vi "Parse_Raw_Response_HTTP.vi"(8 "error in (no error)":errorcluster, 11 "HTTP Response":string) -> (0 "error out":errorcluster, 1 "Headers":cluster{"Name":string, "Value":string}[](array[cluster]), 2 "Status Description":string, 3 "Status Code":string, 4 "Body":string)   [LabVIEW 2016, in "Response.lvclass"]
uses:
  Response.lvclass
panel:
  out "Protocol":string
  out "Status Line":string
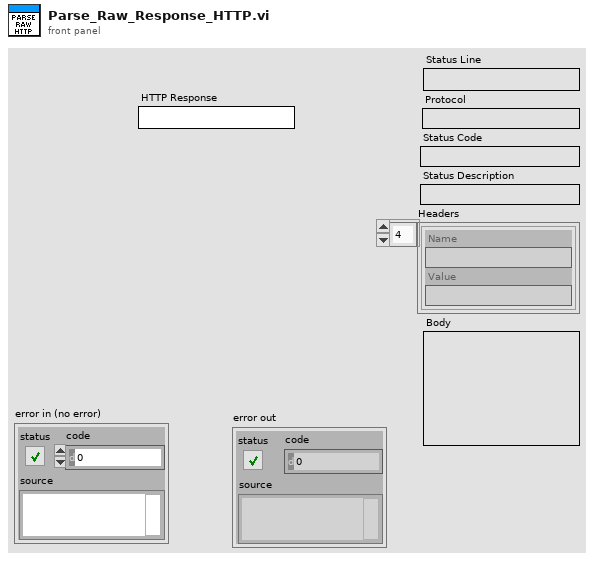
[diagram p1: front panel]
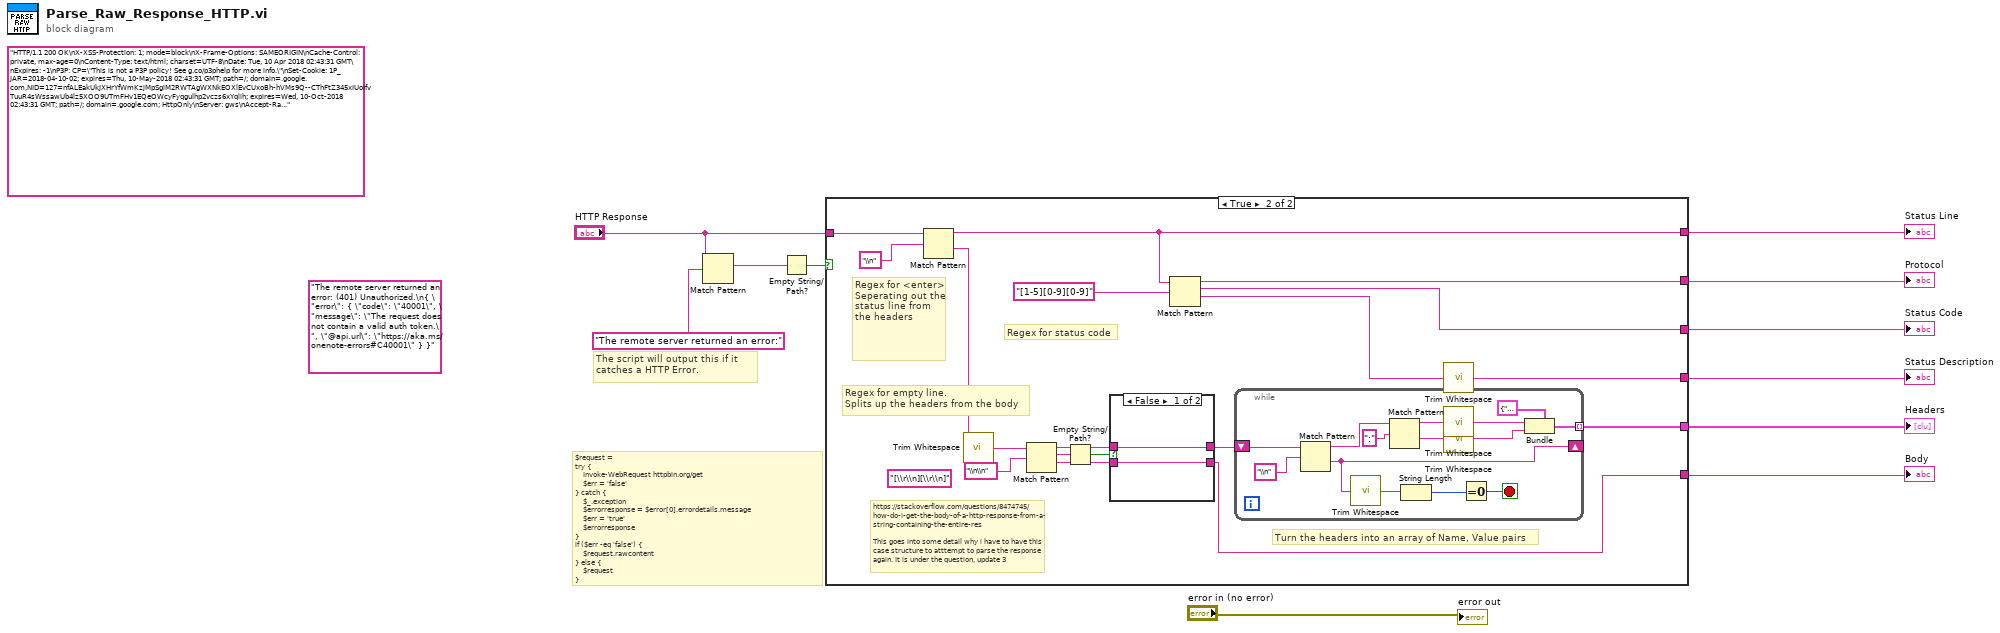
[diagram p0: block diagram]
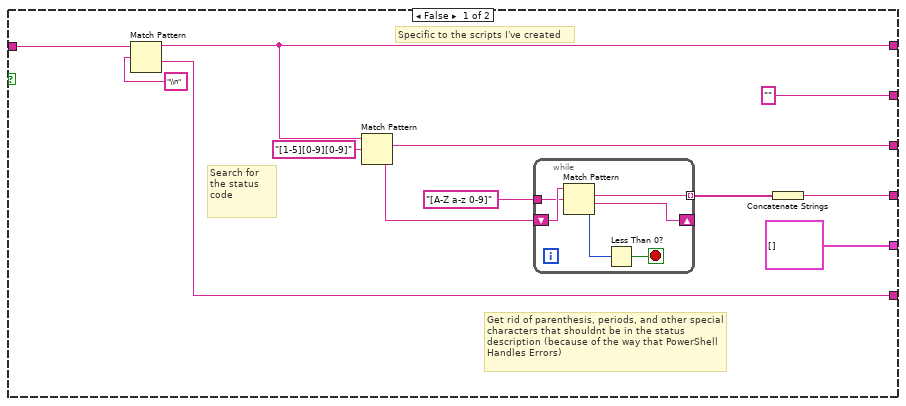
[diagram p2: hidden frame]
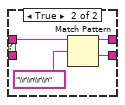
[diagram p3: hidden frame]
diagram:
  (unwired) "The remote server returned an error: (401) Unauthorized.\n{ \"error\": { \"code\": \"40001\", \"message\": \"The request does not contain a valid auth token.\", \"@api.url\": \"https://aka.ms/onenote-errors#C40001\" } }" ("string")
  (unwired) "HTTP/1.1 200 OK\nX-XSS-Protection: 1; mode=block\nX-Frame-Options: SAMEORIGIN\nCache-Control: private, max-age=0\nContent-Type: text/html; charset=UTF-8\nDate: Tue, 10 Apr 2018 02:43:31 GMT\nExpires: -1\nP3P: CP=\"This is not a P3P policy! See g.co/p3phelp for more info.\"\nSet-Cookie: 1P_JAR=2018-04-10-02; expires=Thu, 10-May-2018 02:43:31 GMT; path=/; domain=.google.com,NID=127=nfALEakUkJXHrYfWmKzjMpSgiM2RWTAgWXNkEOXlEvCUxoBh-hVMs9Q--CThFtZ345xIUoIfvTuuR4sWssawUb4lz5XOO9UTmFHv1EQeOWcyFyqgulhp2vczs6xYqlih; expires=Wed, 10-Oct-2018 02:43:31 GMT; path=/; domain=.google.com; HttpOnly\nServer: gws\nAccept-Ranges: none\nVary: Accept-Encoding\nTransfer-Encoding: chunked\n\n<!doctype html><html itemscope=\"\" itemtype=\"http://schema.org/WebPage\" lang=\"en\"><head><meta content=\"Search the world's information, including webpages, images, videos and more. Google has many special features to help you find exactly what you're looking for.\" name=\"description\"><meta content=\"noodp\" name=\"robots\"><meta content=\"text/html; charset=UTF-8\" http-equiv=\"Content-Type\"><meta content=\"/images/branding/googleg/1x/googleg_standard_color_128dp.png\" itemprop=\"image\"><title>Google</title><script nonce=\"MZUWGwd3D7nfH+HpDr55WA==\">(function(){window.google={kEI:'0yTMWqbzMKye_Qam8bXIDw',kEXPI:'0,18167,1335579,530,640,542,217,86,679,339,17,58,365,718,175,4,105,6,50,123,25,216,2341657,142,49,32,302989,26305,1294,12383,2349,2506,32691,16115,317,452,7,792,7,7357,1829,1402,6381,3101,234,2,2,1624,515,4662,364,553,332,332,326,1776,113,1149,465,587,1675,884,632,224,843,1369,136,49,81,3980,208,919,444,354,340,353,200,2,331,230,373,24,287,64,310,296,438,151,467,402,43,325,36,22,2,1,3,276,409,612,388,789,491,71,1694,6,33,121,421,309,129,294,840,352,2,49,430,38,7,1,2,319,242,42,7,636,10,139,166,18,22,191,770,66,195,723,129,8,8,433,490,580,195,5,412,43,224,55,2,435,324,2,107,256,596,327,208,101,56,32,112,234,25,10,428,337,289,138,46,55,2346927,192,4,68,79,7,3686462,12,2533,9,8797651,135,4,1572,549,332,441,2,2,1,2,1,1,77,1,1,900,207,1,1,1,1,1,371,9,438,23,105,4,13,13,8,13,22311637',authuser:0,kscs:'c9c918f0_0yTMWqbzMKye_Qam8bXIDw',u:'c9c918f0',kGL:'US'};google.kHL='en';})();(function(){google.lc=[];google.li=0;google.getEI=function(a){for(var b;a&&(!a.getAttribute||!(b=a.getAttribute(\"eid\")));)a=a.parentNode;return b||google.kEI};google.getLEI=function(a){for(var b=null;a&&(!a.getAttribute||!(b=a.getAttribute(\"leid\")));)a=a.parentNode;return b};google.https=function(){return\"https:\"==window.location.protocol};google.ml=function(){return null};google.wl=function(a,b){try{google.ml(Error(a),!1,b)}catch(d){}};google.time=function(){return(new Date).getTime()};google.log=function(a,b,d,c,g){if(a=google.logUrl(a,b,d,c,g)){b=new Image;var e=google.lc,f=google.li;e[f]=b;b.onerror=b.onload=b.onabort=function(){delete e[f]};google.vel&&google.vel.lu&&google.vel.lu(a);b.src=a;google.li=f+1}};google.logUrl=function(a,b,d,c,g){var e=\"\",f=google.ls||\"\";d||-1!=b.search(\"&ei=\")||(e=\"&ei=\"+google.getEI(c),-1==b.search(\"&lei=\")&&(c=google.getLEI(c))&&(e+=\"&lei=\"+c));c=\"\";!d&&google.cshid&&-1==b.search(\"&cshid=\")&&(c=\"&cshid=\"+google.cshid);a=d||\"/\"+(g||\"gen_204\")+\"?atyp=i&ct=\"+a+\"&cad=\"+b+e+f+\"&zx=\"+google.time()+c;/^http:/i.test(a)&&google.https()&&(google.ml(Error(\"a\"),!1,{src:a,glmm:1}),a=\"\");return a};}).call(this);(function(){google.y={};google.x=function(a,b){if(a)var c=a.id;else{do c=Math.random();while(google.y[c])}google.y[c]=[a,b];return!1};google.lm=[];google.plm=function(a){google.lm.push.apply(google.lm,a)};google.lq=[];google.load=function(a,b,c){google.lq.push([[a],b,c])};google.loadAll=function(a,b){google.lq.push([a,b])};}).call(this);google.f={};var a=window.location,b=a.href.indexOf(\"#\");if(0<=b){var c=a.href.substring(b+1);/(^|&)q=/.test(c)&&-1==c.indexOf(\"#\")&&a.replace(\"/search?\"+c.replace(/(^|&)fp=[^&]*/g,\"\")+\"&cad=h\")};</script><style>#gb{font:13px/27px Arial,sans-serif;height:30px}#gbz,#gbg{position:absolute;white-space:nowrap;top:0;height:30px;z-index:1000}#gbz{left:0;padding-left:4px}#gbg{right:0;padding-right:5px}#gbs{background:transparent;position:absolute;top:-999px;visibility:hidden;z-index:998;right:0}.gbto #gbs{background:#fff}#gbx3,#gbx4{background-color:#2d2d2d;background-image:none;_background-image:none;background-position:0 -138px;background-repeat:repeat-x;border-bottom:1px solid #000;font-size:24px;height:29px;_height:30px;opacity:1;filter:alpha(opacity=100);position:absolute;top:0;width:100%;z-index:990}#gbx3{left:0}#gbx4{right:0}#gbb{position:relative}#gbbw{left:0;position:absolute;top:30px;width:100%}.gbtcb{position:absolute;visibility:hidden}#gbz .gbtcb{right:0}#gbg .gbtcb{left:0}.gbxx{display:none !important}.gbxo{opacity:0 !important;filter:alpha(opacity=0) !important}.gbm{position:absolute;z-index:999;top:-999px;visibility:hidden;text-align:left;border:1px solid #bebebe;background:#fff;-moz-box-shadow:-1px 1px 1px rgba(0,0,0,.2);-webkit-box-shadow:0 2px 4px rgba(0,0,0,.2);box-shadow:0 2px 4px rgba(0,0,0,.2)}.gbrtl .gbm{-moz-box-shadow:1px 1px 1px rgba(0,0,0,.2)}.gbto .gbm,.gbto #gbs{top:29px;visibility:visible}#gbz .gbm{left:0}#gbg .gbm{right:0}.gbxms{background-color:#ccc;display:block;position:absolute;z-index:1;top:-1px;left:-2px;right:-2px;bottom:-2px;opacity:.4;-moz-border-radius:3px;filter:progid:DXImageTransform.Microsoft.Blur(pixelradius=5);*opacity:1;*top:-2px;*left:-5px;*right:5px;*bottom:4px;-ms-filter:\"progid:DXImageTransform.Microsoft.Blur(pixelradius=5)\";opacity:1\\0/;top:-4px\\0/;left:-6px\\0/;right:5px\\0/;bottom:4px\\0/}.gbma{position:relative;top:-1px;border-style:solid dashed dashed;border-color:transparent;border-top-color:#c0c0c0;display:-moz-inline-box;display:inline-block;font-size:0;height:0;line-height:0;width:0;border-width:3px 3px 0;padding-top:1px;left:4px}#gbztms1,#gbi4m1,#gbi4s,#gbi4t{zoom:1}.gbtc,.gbmc,.gbmcc{display:block;list-style:none;margin:0;padding:0}.gbmc{background:#fff;padding:10px 0;position:relative;z-index:2;zoom:1}.gbt{position:relative;display:-moz-inline-box;display:inline-block;line-height:27px;padding:0;vertical-align:top}.gbt{*display:inline}.gbto{box-shadow:0 2px 4px rgba(0,0,0,.2);-moz-box-shadow:0 2px 4px rgba(0,0,0,.2);-webkit-box-shadow:0 2px 4px rgba(0,0,0,.2)}.gbzt,.gbgt{cursor:pointer;display:block;text-decoration:none !important}span#gbg6,span#gbg4{cursor:default}.gbts{border-left:1px solid transparent;border-right:1px solid transparent;display:block;*display:inline-block;padding:0 5px;position:relative;z-index:1000}.gbts{*display:inline}.gbzt .gbts{display:inline;zoom:1}.gbto .gbts{background:#fff;border-color:#bebebe;color:#36c;padding-bottom:1px;padding-top:2px}.gbz0l .gbts{color:#fff;font-weight:bold}.gbtsa{padding-right:9px}#gbz .gbzt,#gbz .gbgt,#gbg .gbgt{color:#ccc!important}.gbtb2{display:block;border-top:2px solid transparent}.gbto .gbzt .gbtb2,.gbto .gbgt .gbtb2{border-top-width:0}.gbtb .gbts{background:url(https://ssl.gstatic.com/gb/images/b_8d5afc09.png);_background:url(https://ssl.gstatic.com/gb/images/b8_3615d64d.png);background-position:-27px -22px;border:0;font-size:0;padding:29px 0 0;*padding:27px 0 0;width:1px}.gbzt:hover,.gbzt:focus,.gbgt-hvr,.gbgt:focus{background-color:#4c4c4c;background-image:none;_background-image:none;background-position:0 -102px;background-repeat:repeat-x;outline:none;text-decoration:none !important}.gbpdjs .gbto .gbm{min-width:99%}.gbz0l .gbtb2{border-top-color:#dd4b39!important}#gbi4s,#gbi4s1{font-weight:bold}#gbg6.gbgt-hvr,#gbg6.gbgt:focus{background-color:transparent;background-image:none}.gbg4a{font-size:0;line-height:0}.gbg4a .gbts{padding:27px 5px 0;*padding:25px 5px 0}.gbto .gbg4a .gbts{padding:29px 5px 1px;*padding:27px 5px 1px}#gbi4i,#gbi4id{left:5px;border:0;height:24px;position:absolute;top:1px;width:24px}.gbto #gbi4i,.gbto #gbi4id{top:3px}.gbi4p{display:block;width:24px}#gbi4id{background-position:-44px -101px}#gbmpid{background-position:0 0}#gbmpi,#gbmpid{border:none;display:inline-block;height:48px;width:48px}#gbmpiw{display:inline-block;line-height:9px;padding-left:20px;margin-top:10px;position:relative}#gbmpi,#gbmpid,#gbmpiw{*display:inline}#gbg5{font-size:0}#gbgs5{padding:5px !important}.gbto #gbgs5{padding:7px 5px 6px !important}#gbi5{background:url(https://ssl.gstatic.com/gb/images/b_8d5afc09.png);_background:url(https://ssl.gstatic.com/gb/images/b8_3615d64d.png);background-position:0 0;display:block;font-size:0;height:17px;width:16px}.gbto #gbi5{background-position:-6px -22px}.gbn .gbmt,.gbn .gbmt:visited,.gbnd .gbmt,.gbnd .gbmt:visited{color:#dd8e27 !important}.gbf .gbmt,.gbf .gbmt:visited{color:#900 !important}.gbmt,.gbml1,.gbmlb,.gbmt:visited,.gbml1:visited,.gbmlb:visited{color:#36c !important;text-decoration:none !important}.gbmt,.gbmt:visited{display:block}.gbml1,.gbmlb,.gbml1:visited,.gbmlb:visited{display:inline-block;margin:0 10px}.gbml1,.gbmlb,.gbml1:visited,.gbmlb:visited{*display:inline}.gbml1,.gbml1:visited{padding:0 10px}.gbml1-hvr,.gbml1:focus{outline:none;text-decoration:underline !important}#gbpm .gbml1{display:inline;margin:0;padding:0;white-space:nowrap}.gbmlb,.gbmlb:visited{line-height:27px}.gbmlb-hvr,.gbmlb:focus{outline:none;text-decoration:underline !important}.gbmlbw{color:#ccc;margin:0 10px}.gbmt{padding:0 20px}.gbmt:hover,.gbmt:focus{background:#eee;cursor:pointer;outline:0 solid black;text-decoration:none !important}.gbm0l,.gbm0l:visited{color:#000 !important;font-weight:bold}.gbmh{border-top:1px solid #bebebe;font-size:0;margin:10px 0}#gbd4 .gbmc{background:#f5f5f5;padding-top:0}#gbd4 .gbsbic::-webkit-scrollbar-track:vertical{background-color:#f5f5f5;margin-top:2px}#gbmpdv{background:#fff;border-bottom:1px solid #bebebe;-moz-box-shadow:0 2px 4px rgba(0,0,0,.12);-o-box-shadow:0 2px 4px rgba(0,0,0,.12);-webkit-box-shadow:0 2px 4px rgba(0,0,0,.12);box-shadow:0 2px 4px rgba(0,0,0,.12);position:relative;z-index:1}#gbd4 .gbmh{margin:0}.gbmtc{padding:0;margin:0;line-height:27px}.GBMCC:last-child:after,#GBMPAL:last-child:after{content:'\\0A\\0A';white-space:pre;position:absolute}#gbmps{*zoom:1}#gbd4 .gbpc,#gbmpas .gbmt{line-height:17px}#gbd4 .gbpgs .gbmtc{line-height:27px}#gbd4 .gbmtc{border-bottom:1px solid #bebebe}#gbd4 .gbpc{display:inline-block;margin:16px 0 10px;padding-right:50px;vertical-align:top}#gbd4 .gbpc{*display:inline}.gbpc .gbps,.gbpc .gbps2{display:block;margin:0 20px}#gbmplp.gbps{margin:0 10px}.gbpc .gbps{color:#000;font-weight:bold}.gbpc .gbpd{margin-bottom:5px}.gbpd .gbmt,.gbpd .gbps{color:#666 !important}.gbpd .gbmt{opacity:.4;filter:alpha(opacity=40)}.gbps2{color:#666;display:block}.gbp0{display:none}.gbp0 .gbps2{font-weight:bold}#gbd4 .gbmcc{margin-top:5px}.gbpmc{background:#fef9db}.gbpmc .gbpmtc{padding:10px 20px}#gbpm{border:0;*border-collapse:collapse;border-spacing:0;margin:0;white-space:normal}#gbpm .gbpmtc{border-top:none;color:#000 !important;font:11px Arial,sans-serif}#gbpms{*white-space:nowrap}.gbpms2{font-weight:bold;white-space:nowrap}#gbmpal{*border-collapse:collapse;border-spacing:0;border:0;margin:0;white-space:nowrap;width:100%}.gbmpala,.gbmpalb{font:13px Arial,sans-serif;line-height:27px;padding:10px 20px 0;white-space:nowrap}.gbmpala{padding-left:0;text-align:left}.gbmpalb{padding-right:0;text-align:right}#gbmpasb .gbps{color:#000}#gbmpal .gbqfbb{margin:0 20px}.gbp0 .gbps{*display:inline}a.gbiba{margin:8px 20px 10px}.gbmpiaw{display:inline-block;padding-right:10px;margin-bottom:6px;margin-top:10px}.gbxv{visibility:hidden}.gbmpiaa{display:block;margin-top:10px}.gbmpia{border:none;display:block;height:48px;width:48px}.gbmpnw{display:inline-block;height:auto;margin:10px 0;vertical-align:top}\n.gbqfb,.gbqfba,.gbqfbb{-moz-border-radius:2px;-webkit-border-radius:2px;border-radius:2px;cursor:default !important;display:inline-block;font-weight:bold;height:29px;line-height:29px;min-width:54px;*min-width:70px;padding:0 8px;text-align:center;text-decoration:none !important;-moz-user-select:none;-webkit-user-select:none}.gbqfb:focus,.gbqfba:focus,.gbqfbb:focus{border:1px solid #4d90fe;-moz-box-shadow:inset 0 0 0 1px rgba(255, 255, 255, 0.5);-webkit-box-shadow:inset 0 0 0 1px rgba(255, 255, 255, 0.5);box-shadow:inset 0 0 0 1px rgba(255, 255, 255, 0.5);outline:none}.gbqfb-hvr:focus,.gbqfba-hvr:focus,.gbqfbb-hvr:focus{-webkit-box-shadow:inset 0 0 0 1px #fff,0 1px 1px rgba(0,0,0,.1);-moz-box-shadow:inset 0 0 0 1px #fff,0 1px 1px rgba(0,0,0,.1);box-shadow:inset 0 0 0 1px #fff,0 1px 1px rgba(0,0,0,.1)}.gbqfb-no-focus:focus{border:1px solid #3079ed;-moz-box-shadow:none;-webkit-box-shadow:none;box-shadow:none}.gbqfb-hvr,.gbqfba-hvr,.gbqfbb-hvr{-webkit-box-shadow:0 1px 1px rgba(0,0,0,.1);-moz-box-shadow:0 1px 1px rgba(0,0,0,.1);box-shadow:0 1px 1px rgba(0,0,0,.1)}.gbqfb::-moz-focus-inner,.gbqfba::-moz-focus-inner,.gbqfbb::-moz-focus-inner{border:0}.gbqfba,.gbqfbb{border:1px solid #dcdcdc;border-color:rgba(0,0,0,.1);color:#444 !important;font-size:11px}.gbqfb{background-color:#4d90fe;background-image:-webkit-gradient(linear,left top,left bottom,from(#4d90fe),to(#4787ed));background-image:-webkit-linear-gradient(top,#4d90fe,#4787ed);background-image:-moz-linear-gradient(top,#4d90fe,#4787ed);background-image:-ms-linear-gradient(top,#4d90fe,#4787ed);background-image:-o-linear-gradient(top,#4d90fe,#4787ed);background-image:linear-gradient(top,#4d90fe,#4787ed);filter:progid:DXImageTransform.Microsoft.gradient(startColorStr='#4d90fe',EndColorStr='#4787ed');border:1px solid #3079ed;color:#fff!important;margin:0 0}.gbqfb-hvr{border-color:#2f5bb7}.gbqfb-hvr:focus{border-color:#2f5bb7}.gbqfb-hvr,.gbqfb-hvr:focus{background-color:#357ae8;background-image:-webkit-gradient(linear,left top,left bottom,from(#4d90fe),to(#357ae8));background-image:-webkit-linear-gradient(top,#4d90fe,#357ae8);background-image:-moz-linear-gradient(top,#4d90fe,#357ae8);background-image:-ms-linear-gradient(top,#4d90fe,#357ae8);background-image:-o-linear-gradient(top,#4d90fe,#357ae8);background-image:linear-gradient(top,#4d90fe,#357ae8)}.gbqfb:active{background-color:inherit;-webkit-box-shadow:inset 0 1px 2px rgba(0, 0, 0, 0.3);-moz-box-shadow:inset 0 1px 2px rgba(0, 0, 0, 0.3);box-shadow:inset 0 1px 2px rgba(0, 0, 0, 0.3)}.gbqfba{background-color:#f5f5f5;background-image:-webkit-gradient(linear,left top,left bottom,from(#f5f5f5),to(#f1f1f1));background-image:-webkit-linear-gradient(top,#f5f5f5,#f1f1f1);background-image:-moz-linear-gradient(top,#f5f5f5,#f1f1f1);background-image:-ms-linear-gradient(top,#f5f5f5,#f1f1f1);background-image:-o-linear-gradient(top,#f5f5f5,#f1f1f1);background-image:linear-gradient(top,#f5f5f5,#f1f1f1);filter:progid:DXImageTransform.Microsoft.gradient(startColorStr='#f5f5f5',EndColorStr='#f1f1f1')}.gbqfba-hvr,.gbqfba-hvr:active{background-color:#f8f8f8;background-image:-webkit-gradient(linear,left top,left bottom,from(#f8f8f8),to(#f1f1f1));background-image:-webkit-linear-gradient(top,#f8f8f8,#f1f1f1);background-image:-moz-linear-gradient(top,#f8f8f8,#f1f1f1);background-image:-ms-linear-gradient(top,#f8f8f8,#f1f1f1);background-image:-o-linear-gradient(top,#f8f8f8,#f1f1f1);background-image:linear-gradient(top,#f8f8f8,#f1f1f1);filter:progid:DXImageTransform.Microsoft.gradient(startColorStr='#f8f8f8',EndColorStr='#f1f1f1')}.gbqfbb{background-color:#fff;background-image:-webkit-gradient(linear,left top,left bottom,from(#fff),to(#fbfbfb));background-image:-webkit-linear-gradient(top,#fff,#fbfbfb);background-image:-moz-linear-gradient(top,#fff,#fbfbfb);background-image:-ms-linear-gradient(top,#fff,#fbfbfb);background-image:-o-linear-gradient(top,#fff,#fbfbfb);background-image:linear-gradient(top,#fff,#fbfbfb);filter:progid:DXImageTransform.Microsoft.gradient(startColorStr='#ffffff',EndColorStr='#fbfbfb')}.gbqfbb-hvr,.gbqfbb-hvr:active{background-color:#fff;background-image:-webkit-gradient(linear,left top,left bottom,from(#fff),to(#f8f8f8));background-image:-webkit-linear-gradient(top,#fff,#f8f8f8);background-image:-moz-linear-gradient(top,#fff,#f8f8f8);background-image:-ms-linear-gradient(top,#fff,#f8f8f8);background-image:-o-linear-gradient(top,#fff,#f8f8f8);background-image:linear-gradient(top,#fff,#f8f8f8);filter:progid:DXImageTransform.Microsoft.gradient(startColorStr='#ffffff',EndColorStr='#f8f8f8')}.gbqfba-hvr,.gbqfba-hvr:active,.gbqfbb-hvr,.gbqfbb-hvr:active{border-color:#c6c6c6;-webkit-box-shadow:0 1px 1px rgba(0,0,0,.1);-moz-box-shadow:0 1px 1px rgba(0,0,0,.1);box-shadow:0 1px 1px rgba(0,0,0,.1);color:#222 !important}.gbqfba:active,.gbqfbb:active{-webkit-box-shadow:inset 0 1px 2px rgba(0,0,0,.1);-moz-box-shadow:inset 0 1px 2px rgba(0,0,0,.1);box-shadow:inset 0 1px 2px rgba(0,0,0,.1)}\n#gbmpas{max-height:220px}#gbmm{max-height:530px}.gbsb{-webkit-box-sizing:border-box;display:block;position:relative;*zoom:1}.gbsbic{overflow:auto}.gbsbis .gbsbt,.gbsbis .gbsbb{-webkit-mask-box-image:-webkit-gradient(linear,left top,right top,color-stop(0,rgba(0,0,0,.1)),color-stop(.5,rgba(0,0,0,.8)),color-stop(1,rgba(0,0,0,.1)));left:0;margin-right:0;opacity:0;position:absolute;width:100%}.gbsb .gbsbt:after,.gbsb .gbsbb:after{content:\"\";display:block;height:0;left:0;position:absolute;width:100%}.gbsbis .gbsbt{background:-webkit-gradient(linear,left top,left bottom,from(rgba(0,0,0,.2)),to(rgba(0,0,0,0)));background-image:-webkit-linear-gradient(top,rgba(0,0,0,.2),rgba(0,0,0,0));background-image:-moz-linear-gradient(top,rgba(0,0,0,.2),rgba(0,0,0,0));background-image:-ms-linear-gradient(top,rgba(0,0,0,.2),rgba(0,0,0,0));background-image:-o-linear-gradient(top,rgba(0,0,0,.2),rgba(0,0,0,0));background-image:linear-gradient(top,rgba(0,0,0,.2),rgba(0,0,0,0));height:6px;top:0}.gbsb .gbsbt:after{border-top:1px solid #ebebeb;border-color:rgba(0,0,0,.3);top:0}.gbsb .gbsbb{-webkit-mask-box-image:-webkit-gradient(linear,left top,right top,color-stop(0,rgba(0,0,0,.1)),color-stop(.5,rgba(0,0,0,.8)),color-stop(1,rgba(0,0,0,.1)));background:-webkit-gradient(linear,left bottom,left top,from(rgba(0,0,0,.2)),to(rgba(0,0,0,0)));background-image:-webkit-linear-gradient(bottom,rgba(0,0,0,.2),rgba(0,0,0,0));background-image:-moz-linear-gradient(bottom,rgba(0,0,0,.2),rgba(0,0,0,0));background-image:-ms-linear-gradient(bottom,rgba(0,0,0,.2),rgba(0,0,0,0));background-image:-o-linear-gradient(bottom,rgba(0,0,0,.2),rgba(0,0,0,0));background-image:linear-gradient(bottom,rgba(0,0,0,.2),rgba(0,0,0,0));bottom:0;height:4px}.gbsb .gbsbb:after{border-bottom:1px solid #ebebeb;border-color:rgba(0,0,0,.3);bottom:0}\n</style><style>body,td,a,p,.h{font-family:arial,sans-serif}body{margin:0;overflow-y:scroll}#gog{padding:3px 8px 0}td{line-height:.8em}.gac_m td{line-height:17px}form{margin-bottom:20px}.h{color:#36c}.q{color:#00c}.ts td{padding:0}.ts{border-collapse:collapse}em{font-weight:bold;font-style:normal}.lst{height:25px;width:496px}.gsfi,.lst{font:18px arial,sans-serif}.gsfs{font:17px arial,sans-serif}.ds{display:inline-box;display:inline-block;margin:3px 0 4px;margin-left:4px}input{font-family:inherit}a.gb1,a.gb2,a.gb3,a.gb4{color:#11c !important}body{background:#fff;color:black}a{color:#11c;text-decoration:none}a:hover,a:active{text-decoration:underline}.fl a{color:#36c}a:visited{color:#551a8b}a.gb1,a.gb4{text-decoration:underline}a.gb3:hover{text-decoration:none}#ghead a.gb2:hover{color:#fff !important}.sblc{padding-top:5px}.sblc a{display:block;margin:2px 0;margin-left:13px;font-size:11px}.lsbb{background:#eee;border:solid 1px;border-color:#ccc #999 #999 #ccc;height:30px}.lsbb{display:block}.ftl,#fll a{display:inline-block;margin:0 12px}.lsb{background:url(/images/nav_logo229.png) 0 -261px repeat-x;border:none;color:#000;cursor:pointer;height:30px;margin:0;outline:0;font:15px arial,sans-serif;vertical-align:top}.lsb:active{background:#ccc}.lst:focus{outline:none}</style><script nonce=\"MZUWGwd3D7nfH+HpDr55WA==\">(function(){try{var e=this;var aa=function(a,b,c,d){d=d||{};d._sn=[\"cfg\",b,c].join(\".\");window.gbar.logger.ml(a,d)};var g=window.gbar=window.gbar||{},h=window.gbar.i=window.gbar.i||{},ba;function _tvn(a,b){a=parseInt(a,10);return isNaN(a)?b:a}function _tvf(a,b){a=parseFloat(a);return isNaN(a)?b:a}function _tvv(a){return!!a}function p(a,b,c){(c||g)[a]=b}g.bv={n:_tvn(\"2\",0),r:\"\",f:\".66.41.\",e:\"1300102,3700298,3700440,3700489,3700521\",m:_tvn(\"1\",1)};\nfunction ca(a,b,c){var d=\"on\"+b;if(a.addEventListener)a.addEventListener(b,c,!1);else if(a.attachEvent)a.attachEvent(d,c);else{var f=a[d];a[d]=function(){var a=f.apply(this,arguments),b=c.apply(this,arguments);return void 0==a?b:void 0==b?a:b&&a}}}var da=function(a){return function(){return g.bv.m==a}},ea=da(1),fa=da(2);p(\"sb\",ea);p(\"kn\",fa);h.a=_tvv;h.b=_tvf;h.c=_tvn;h.i=aa;var q=window.gbar.i.i;var r=function(){},ha=function(){},ka=function(a){var b=new Image,c=ia;b.onerror=b.onload=b.onabort=function(){try{delete ja[c]}catch(d){}};ja[c]=b;b.src=a;ia=c+1},ja=[],ia=0;p(\"logger\",{il:ha,ml:r,log:ka});var u=window.gbar.logger;var v={},la={},w=[],ma=h.b(\"0.1\",.1),na=h.a(\"1\",!0),oa=function(a,b){w.push([a,b])},pa=function(a,b){v[a]=b},qa=function(a){return a in v},x={},A=function(a,b){x[a]||(x[a]=[]);x[a].push(b)},B=function(a){A(\"m\",a)},ra=function(a,b){var c=document.createElement(\"script\");c.src=a;c.async=na;Math.random()<ma&&(c.onerror=function(){c.onerror=null;r(Error(\"Bundle load failed: name=\"+(b||\"UNK\")+\" url=\"+a))});(document.getElementById(\"xjsc\")||document.getElementsByTagName(\"body\")[0]||\ndocument.getElementsByTagName(\"head\")[0]).appendChild(c)},D=function(a){for(var b=0,c;(c=w[b])&&c[0]!=a;++b);!c||c[1].l||c[1].s||(c[1].s=!0,sa(2,a),c[1].url&&ra(c[1].url,a),c[1].libs&&C&&C(c[1].libs))},ta=function(a){A(\"gc\",a)},ua=null,va=function(a){ua=a},sa=function(a,b,c){if(ua){a={t:a,b:b};if(c)for(var d in c)a[d]=c[d];try{ua(a)}catch(f){}}};p(\"mdc\",v);p(\"mdi\",la);p(\"bnc\",w);p(\"qGC\",ta);p(\"qm\",B);p(\"qd\",x);p(\"lb\",D);p(\"mcf\",pa);p(\"bcf\",oa);p(\"aq\",A);p(\"mdd\",\"\");\np(\"has\",qa);p(\"trh\",va);p(\"tev\",sa);if(h.a(\"m;/_/scs/abc-static/_/js/k=gapi.gapi.en.wjAGE-AVlTo.O/m=__features__/am=AAE/rt=j/d=1/rs=AHpOoo-gY863zTybf8wCUIW8gIU8UfC49g\")){var F=function(a,b){return wa?a||b:b},xa=h.a(\"1\"),ya=h.a(\"\"),za=h.a(\"\"),wa=h.a(\"\"),Aa=window.gapi=F(window.gapi,{}),Ba=function(a,b){var c=function(){g.dgl(a,b)};xa?B(c):(A(\"gl\",c),D(\"gl\"))},Ca={},Da=function(a){a=a.split(\":\");for(var b;(b=a.pop())&&Ca[b];);return!b},C=function(a){function b(){for(var b=a.split(\":\"),d=0,f;f=b[d];++d)Ca[f]=1;for(b=0;d=w[b];++b)d=d[1],(f=d.libs)&&!d.l&&d.i&&\nDa(f)&&d.i()}g.dgl(a,b)},G=window.___jsl=F(window.___jsl,{});G.h=F(G.h,\"m;/_/scs/abc-static/_/js/k=gapi.gapi.en.wjAGE-AVlTo.O/m=__features__/am=AAE/rt=j/d=1/rs=AHpOoo-gY863zTybf8wCUIW8gIU8UfC49g\");G.ms=F(G.ms,\"https://apis.google.com\");G.m=F(G.m,\"\");G.l=F(G.l,[]);xa||w.push([\"gl\",{url:\"//ssl.gstatic.com/gb/js/abc/glm_e7bb39a7e1a24581ff4f8d199678b1b9.js\"}]);var Ea={pu:ya,sh:\"\",si:za,hl:\"en\"};v.gl=Ea;wa?Aa.load||p(\"load\",Ba,Aa):p(\"load\",Ba,Aa);p(\"dgl\",Ba);p(\"agl\",Da);h.o=xa};var Fa=h.b(\"0.1\",.001),Ga=0;\nfunction _mlToken(a,b){try{if(1>Ga){Ga++;var c=a;b=b||{};var d=encodeURIComponent,f=[\"//www.google.com/gen_204?atyp=i&zx=\",(new Date).getTime(),\"&jexpid=\",d(\"28834\"),\"&srcpg=\",d(\"prop=1\"),\"&jsr=\",Math.round(1/Fa),\"&ogev=\",d(\"0yTMWv3UMeGN_QaribqQCQ\"),\"&ogf=\",g.bv.f,\"&ogrp=\",d(\"\"),\"&ogv=\",d(\"190405948.0\"),\"&oggv=\"+d(\"es_plusone_gc_20180321.0_p0\"),\"&ogd=\",d(\"com\"),\"&ogc=\",d(\"USA\"),\"&ogl=\",d(\"en\")];b._sn&&(b._sn=\n\"og.\"+b._sn);for(var k in b)f.push(\"&\"),f.push(d(k)),f.push(\"=\"),f.push(d(b[k]));f.push(\"&emsg=\");f.push(d(c.name+\":\"+c.message));var l=f.join(\"\");Ha(l)&&(l=l.substr(0,2E3));var m=l;var n=window.gbar.logger._aem(a,m);ka(n)}}catch(t){}}var Ha=function(a){return 2E3<=a.length},Ia=function(a,b){return b};function Ja(a){r=a;p(\"_itl\",Ha,u);p(\"_aem\",Ia,u);p(\"ml\",r,u);a={};v.er=a}h.a(\"\")?Ja(function(a){throw a;}):h.a(\"1\")&&Math.random()<Fa&&Ja(_mlToken);var _E=\"left\",Ka=h.a(\"\"),J=function(a,b){var c=a.className;H(a,b)||(a.className+=(\"\"!=c?\" \":\"\")+b)},K=function(a,b){var c=a.className;b=new RegExp(\"\\\\s?\\\\b\"+b+\"\\\\b\");c&&c.match(b)&&(a.className=c.replace(b,\"\"))},H=function(a,b){b=new RegExp(\"\\\\b\"+b+\"\\\\b\");a=a.className;return!(!a||!a.match(b))},La=function(a,b){H(a,b)?K(a,b):J(a,b)},Ma=function(a,b){a[b]=function(c){var d=arguments;g.qm(function(){a[b].apply(this,d)})}},Na=function(){return\"1\"},\nOa=function(a){a=[\"//www.gstatic.com\",\"/og/_/js/d=1/k=\",\"og.og2.en_US.DsHOofbGMmQ.O\",\"/rt=j/m=\",a,\"/rs=\",\"AA2YrTunYyhQXRvVKqTSwejvoR73Wu4Flw\"];Ka&&a.push(\"?host=www.gstatic.com&bust=og.og2.en_US.N2cSruH95IY.DU\");a=a.join(\"\");ra(a)};p(\"ca\",J);p(\"cr\",K);p(\"cc\",H);h.k=J;h.l=K;h.m=H;h.n=La;h.p=Oa;h.q=Ma;h.r=Na;var Pa=[\"gb_71\",\"gb_155\"],Qa;function Ra(a){Qa=a}function Sa(a){var b=Qa&&!a.href.match(/.*\\/accounts\\/ClearSID[?]/)&&encodeURIComponent(Qa());b&&(a.href=a.href.replace(/([?&]continue=)[^&]*/,\"$1\"+b))}function Ta(a){window.gApplication&&(a.href=window.gApplication.getTabUrl(a.href))}function Ua(a){try{var b=(document.forms[0].q||\"\").value;b&&(a.href=a.href.replace(/([?&])q=[^&]*|$/,function(a,d){return(d||\"&\")+\"q=\"+encodeURIComponent(b)}))}catch(c){q(c,\"sb\",\"pq\")}}\nvar Va=function(){for(var a=[],b=0,c;c=Pa[b];++b)(c=document.getElementById(c))&&a.push(c);return a},Wa=function(){var a=Va();return 0<a.length?a[0]:null},Xa=function(){return document.getElementById(\"gb_70\")},L={},M={},Ya={},N={},O=void 0,cb=function(a,b){try{var c=document.getElementById(\"gb\");J(c,\"gbpdjs\");P();Za(document.getElementById(\"gb\"))&&J(c,\"gbrtl\");if(b&&b.getAttribute){var d=b.getAttribute(\"aria-owns\");if(d.length){var f=document.getElementById(d);if(f){var k=b.parentNode;if(O==d)O=void 0,\nK(k,\"gbto\");else{if(O){var l=document.getElementById(O);if(l&&l.getAttribute){var m=l.getAttribute(\"aria-owner\");if(m.length){var n=document.getElementById(m);n&&n.parentNode&&K(n.parentNode,\"gbto\")}}}$a(f)&&ab(f);O=d;J(k,\"gbto\")}}}}B(function(){g.tg(a,b,!0)});bb(a)}catch(t){q(t,\"sb\",\"tg\")}},db=function(a){B(function(){g.close(a)})},eb=function(a){B(function(){g.rdd(a)})},Za=function(a){var b,c=document.defaultView;c&&c.getComputedStyle?(a=c.getComputedStyle(a,\"\"))&&(b=a.direction):b=a.currentStyle?\na.currentStyle.direction:a.style.direction;return\"rtl\"==b},gb=function(a,b,c){if(a)try{var d=document.getElementById(\"gbd5\");if(d){var f=d.firstChild,k=f.firstChild,l=document.createElement(\"li\");l.className=b+\" gbmtc\";l.id=c;a.className=\"gbmt\";l.appendChild(a);if(k.hasChildNodes()){c=[[\"gbkc\"],[\"gbf\",\"gbe\",\"gbn\"],[\"gbkp\"],[\"gbnd\"]];d=0;var m=k.childNodes.length;f=!1;for(var n=-1,t=0,E;E=c[t];t++){for(var U=0,I;I=E[U];U++){for(;d<m&&H(k.childNodes[d],I);)d++;if(I==b){k.insertBefore(l,k.childNodes[d]||\nnull);f=!0;break}}if(f){if(d+1<k.childNodes.length){var V=k.childNodes[d+1];H(V.firstChild,\"gbmh\")||fb(V,E)||(n=d+1)}else if(0<=d-1){var W=k.childNodes[d-1];H(W.firstChild,\"gbmh\")||fb(W,E)||(n=d)}break}0<d&&d+1<m&&d++}if(0<=n){var y=document.createElement(\"li\"),z=document.createElement(\"div\");y.className=\"gbmtc\";z.className=\"gbmt gbmh\";y.appendChild(z);k.insertBefore(y,k.childNodes[n])}g.addHover&&g.addHover(a)}else k.appendChild(l)}}catch(Eb){q(Eb,\"sb\",\"al\")}},fb=function(a,b){for(var c=b.length,\nd=0;d<c;d++)if(H(a,b[d]))return!0;return!1},hb=function(a,b,c){gb(a,b,c)},ib=function(a,b){gb(a,\"gbe\",b)},jb=function(){B(function(){g.pcm&&g.pcm()})},kb=function(){B(function(){g.pca&&g.pca()})},lb=function(a,b,c,d,f,k,l,m,n,t){B(function(){g.paa&&g.paa(a,b,c,d,f,k,l,m,n,t)})},mb=function(a,b){L[a]||(L[a]=[]);L[a].push(b)},nb=function(a,b){M[a]||(M[a]=[]);M[a].push(b)},ob=function(a,b){Ya[a]=b},pb=function(a,b){N[a]||(N[a]=[]);N[a].push(b)},bb=function(a){a.preventDefault&&a.preventDefault();a.returnValue=\n!1;a.cancelBubble=!0},qb=null,ab=function(a,b){P();if(a){rb(a,\"Opening&hellip;\");Q(a,!0);b=\"undefined\"!=typeof b?b:1E4;var c=function(){sb(a)};qb=window.setTimeout(c,b)}},tb=function(a){P();a&&(Q(a,!1),rb(a,\"\"))},sb=function(a){try{P();var b=a||document.getElementById(O);b&&(rb(b,\"This service is currently unavailable.%1$sPlease try again later.\",\"%1$s\"),Q(b,!0))}catch(c){q(c,\"sb\",\"sdhe\")}},rb=function(a,b,c){if(a&&b){var d=$a(a);if(d){if(c){d.innerHTML=\"\";b=b.split(c);c=0;for(var f;f=b[c];c++){var k=document.createElement(\"div\");\nk.innerHTML=f;d.appendChild(k)}}else d.innerHTML=b;Q(a,!0)}}},Q=function(a,b){(b=void 0!==b?b:!0)?J(a,\"gbmsgo\"):K(a,\"gbmsgo\")},$a=function(a){for(var b=0,c;c=a.childNodes[b];b++)if(H(c,\"gbmsg\"))return c},P=function(){qb&&window.clearTimeout(qb)},ub=function(a){var b=\"inner\"+a;a=\"offset\"+a;return window[b]?window[b]:document.documentElement&&document.documentElement[a]?document.documentElement[a]:0},vb=function(){return!1},wb=function(){return!!O};p(\"so\",Wa);p(\"sos\",Va);p(\"si\",Xa);p(\"tg\",cb);\np(\"close\",db);p(\"rdd\",eb);p(\"addLink\",hb);p(\"addExtraLink\",ib);p(\"pcm\",jb);p(\"pca\",kb);p(\"paa\",lb);p(\"ddld\",ab);p(\"ddrd\",tb);p(\"dderr\",sb);p(\"rtl\",Za);p(\"op\",wb);p(\"bh\",L);p(\"abh\",mb);p(\"dh\",M);p(\"adh\",nb);p(\"ch\",N);p(\"ach\",pb);p(\"eh\",Ya);p(\"aeh\",ob);ba=h.a(\"\")?Ta:Ua;p(\"qs\",ba);p(\"setContinueCb\",Ra);p(\"pc\",Sa);p(\"bsy\",vb);h.d=bb;h.j=ub;var xb={};v.base=xb;w.push([\"m\",{url:\"//ssl.gstatic.com/gb/js/sem_7e6c732dccf2b05588c7c99408d0d47f.js\"}]);g.sg={c:\"1\"};p(\"wg\",{rg:{}});var yb={tiw:h.c(\"15000\",0),tie:h.c(\"30000\",0)};v.wg=yb;var zb={thi:h.c(\"10000\",0),thp:h.c(\"180000\",0),tho:h.c(\"5000\",0),tet:h.b(\"0.5\",0)};v.wm=zb;if(h.a(\"1\")){var Ab=h.a(\"\");w.push([\"gc\",{auto:Ab,url:\"//ssl.gstatic.com/gb/js/abc/gci_91f30755d6a6b787dcc2a4062e6e9824.js\",libs:\"googleapis.client:plusone:gapi.iframes\"}]);var Bb={version:\"gci_91f30755d6a6b787dcc2a4062e6e9824.js\",index:\"\",lang:\"en\"};v.gc=Bb;var Cb=function(a){window.googleapis&&window.iframes?a&&a():(a&&ta(a),D(\"gc\"))};p(\"lGC\",Cb);h.a(\"1\")&&p(\"lPWF\",Cb)};window.__PVT=\"\";if(h.a(\"1\")&&h.a(\"1\")){var Db=function(a){Cb(function(){A(\"pw\",a);D(\"pw\")})};p(\"lPW\",Db);w.push([\"pw\",{url:\"//ssl.gstatic.com/gb/js/abc/pwm_45f73e4df07a0e388b0fa1f3d30e7280.js\"}]);var Fb=[],Gb=function(a){Fb[0]=a},Hb=function(a,b){b=b||{};b._sn=\"pw\";r(a,b)},Ib={signed:Fb,elog:Hb,base:\"https://plusone.google.com/u/0\",loadTime:(new Date).getTime()};v.pw=Ib;var Jb=function(a,b){var c=b.split(\".\");b=function(){var b=arguments;a(function(){for(var a=g,d=0,f=c.length-1;d<f;++d)a=a[c[d]];a[c[d]].apply(a,b)})};for(var d=g,f=0,k=c.length-1;f<\nk;++f)d=d[c[f]]=d[c[f]]||{};return d[c[f]]=b};Jb(Db,\"pw.clk\");Jb(Db,\"pw.hvr\");p(\"su\",Gb,g.pw)};var Kb=[1,2,3,4,5,6,9,10,11,13,14,28,29,30,34,35,37,38,39,40,41,42,43,48,49,500];var Lb=h.b(\"0.001\",1E-4),Mb=h.b(\"1\",1),Nb=!1,Ob=!1;if(h.a(\"1\")){var Pb=Math.random();Pb<Lb&&(Nb=!0);Pb<Mb&&(Ob=!0)}var R=null;\nfunction Qb(a,b){var c=Lb,d=Nb;var f=a;if(!R){R={};for(var k=0;k<Kb.length;k++){var l=Kb[k];R[l]=!0}}if(f=!!R[f])c=Mb,d=Ob;if(d){d=encodeURIComponent;if(g.rp){var m=g.rp();m=\"-1\"!=m?m:\"\"}else m=\"\";f=(new Date).getTime();k=d(\"28834\");l=d(\"0yTMWv3UMeGN_QaribqQCQ\");var n=g.bv.f,t=d(\"1\");m=d(m);c=Math.round(1/c);var E=d(\"190405948.0\"),U=\"&oggv=\"+d(\"es_plusone_gc_20180321.0_p0\"),I=d(\"com\"),V=d(\"en\"),W=\nd(\"USA\");var y=0;h.a(\"\")&&(y|=1);h.a(\"\")&&(y|=2);h.a(\"\")&&(y|=4);a=[\"//www.google.com/gen_204?atyp=i&zx=\",f,\"&oge=\",a,\"&ogex=\",k,\"&ogev=\",l,\"&ogf=\",n,\"&ogp=\",t,\"&ogrp=\",m,\"&ogsr=\",c,\"&ogv=\",E,U,\"&ogd=\",I,\"&ogl=\",V,\"&ogc=\",W,\"&ogus=\",y];if(b){\"ogw\"in b&&(a.push(\"&ogw=\"+b.ogw),delete b.ogw);f=[];for(z in b)0!=f.length&&f.push(\",\"),f.push(Rb(z)),f.push(\".\"),f.push(Rb(b[z]));var z=f.join(\"\");\"\"!=z&&(a.push(\"&ogad=\"),a.push(d(z)))}ka(a.join(\"\"))}}\nfunction Rb(a){\"number\"==typeof a&&(a+=\"\");return\"string\"==typeof a?a.replace(\".\",\"%2E\").replace(\",\",\"%2C\"):a}ha=Qb;p(\"il\",ha,u);var Sb={};v.il=Sb;var Tb=function(a,b,c,d,f,k,l,m,n,t){B(function(){g.paa(a,b,c,d,f,k,l,m,n,t)})},Ub=function(){B(function(){g.prm()})},Vb=function(a){B(function(){g.spn(a)})},Wb=function(a){B(function(){g.sps(a)})},Xb=function(a){B(function(){g.spp(a)})},Yb={\"27\":\"https://ssl.gstatic.com/gb/images/silhouette_24.png\",\"27\":\"https://ssl.gstatic.com/gb/images/silhouette_24.png\",\"27\":\"https://ssl.gstatic.com/gb/images/silhouette_24.png\"},Zb=function(a){return(a=Yb[a])||\"https://ssl.gstatic.com/gb/images/silhouette_24.png\"},\n$b=function(){B(function(){g.spd()})};p(\"spn\",Vb);p(\"spp\",Xb);p(\"sps\",Wb);p(\"spd\",$b);p(\"paa\",Tb);p(\"prm\",Ub);mb(\"gbd4\",Ub);\nif(h.a(\"\")){var ac={d:h.a(\"\"),e:\"\",sanw:h.a(\"\"),p:\"https://ssl.gstatic.com/gb/images/silhouette_96.png\",cp:\"1\",xp:h.a(\"1\"),mg:\"%1$s (delegated)\",md:\"%1$s (default)\",mh:\"220\",s:\"1\",pp:Zb,ppl:h.a(\"\"),ppa:h.a(\"\"),\nppm:\"Google+ page\"};v.prf=ac};var S,bc,T,cc,X=0,dc=function(a,b,c){if(a.indexOf)return a.indexOf(b,c);if(Array.indexOf)return Array.indexOf(a,b,c);for(c=null==c?0:0>c?Math.max(0,a.length+c):c;c<a.length;c++)if(c in a&&a[c]===b)return c;return-1},Y=function(a,b){return-1==dc(a,X)?(q(Error(X+\"_\"+b),\"up\",\"caa\"),!1):!0},fc=function(a,b){Y([1,2],\"r\")&&(S[a]=S[a]||[],S[a].push(b),2==X&&window.setTimeout(function(){b(ec(a))},0))},gc=function(a,b,c){if(Y([1],\"nap\")&&c){for(var d=0;d<c.length;d++)bc[c[d]]=!0;g.up.spl(a,b,\"nap\",c)}},hc=\nfunction(a,b,c){if(Y([1],\"aop\")&&c){if(T)for(var d in T)T[d]=T[d]&&-1!=dc(c,d);else for(T={},d=0;d<c.length;d++)T[c[d]]=!0;g.up.spl(a,b,\"aop\",c)}},ic=function(){try{if(X=2,!cc){cc=!0;for(var a in S)for(var b=S[a],c=0;c<b.length;c++)try{b[c](ec(a))}catch(d){q(d,\"up\",\"tp\")}}}catch(d){q(d,\"up\",\"mtp\")}},ec=function(a){if(Y([2],\"ssp\")){var b=!bc[a];T&&(b=b&&!!T[a]);return b}};cc=!1;S={};bc={};T=null;X=1;\nvar jc=function(a){var b=!1;try{b=a.cookie&&a.cookie.match(\"PREF\")}catch(c){}return!b},kc=function(){try{return!!e.localStorage&&\"object\"==typeof e.localStorage}catch(a){return!1}},lc=function(a){return a&&a.style&&a.style.behavior&&\"undefined\"!=typeof a.load},mc=function(a,b,c,d){try{jc(document)||(d||(b=\"og-up-\"+b),kc()?e.localStorage.setItem(b,c):lc(a)&&(a.setAttribute(b,c),a.save(a.id)))}catch(f){f.code!=DOMException.QUOTA_EXCEEDED_ERR&&q(f,\"up\",\"spd\")}},nc=function(a,b,c){try{if(jc(document))return\"\";\nc||(b=\"og-up-\"+b);if(kc())return e.localStorage.getItem(b);if(lc(a))return a.load(a.id),a.getAttribute(b)}catch(d){d.code!=DOMException.QUOTA_EXCEEDED_ERR&&q(d,\"up\",\"gpd\")}return\"\"},oc=function(a,b,c){a.addEventListener?a.addEventListener(b,c,!1):a.attachEvent&&a.attachEvent(\"on\"+b,c)},pc=function(a){for(var b=0,c;c=a[b];b++){var d=g.up;c=c in d&&d[c];if(!c)return!1}return!0},qc=function(a,b){try{if(jc(a))return-1;var c=a.cookie.match(/OGPC=([^;]*)/);if(c&&c[1]){var d=c[1].match(new RegExp(\"\\\\b\"+\nb+\"-([0-9]+):\"));if(d&&d[1])return parseInt(d[1],10)}}catch(f){f.code!=DOMException.QUOTA_EXCEEDED_ERR&&q(f,\"up\",\"gcc\")}return-1};p(\"up\",{r:fc,nap:gc,aop:hc,tp:ic,ssp:ec,spd:mc,gpd:nc,aeh:oc,aal:pc,gcc:qc});var Z=function(a,b){a[b]=function(c){var d=arguments;g.qm(function(){a[b].apply(this,d)})}};Z(g.up,\"sl\");Z(g.up,\"si\");Z(g.up,\"spl\");Z(g.up,\"dpc\");Z(g.up,\"iic\");g.mcf(\"up\",{sp:h.b(\"0.01\",1),tld:\"com\",prid:\"1\"});function rc(){function a(){for(var b;(b=k[l++])&&\"m\"!=b[0]&&!b[1].auto;);b&&(sa(2,b[0]),b[1].url&&ra(b[1].url,b[0]),b[1].libs&&C&&C(b[1].libs));l<k.length&&setTimeout(a,0)}function b(){0<f--?setTimeout(b,0):a()}var c=h.a(\"1\"),d=h.a(\"\"),f=3,k=w,l=0,m=window.gbarOnReady;if(m)try{m()}catch(n){q(n,\"ml\",\"or\")}d?p(\"ldb\",a):c?ca(window,\"load\",b):b()}p(\"rdl\",rc);}catch(e){window.gbar&&gbar.logger&&gbar.logger.ml(e,{\"_sn\":\"cfg.init\"});}})();\n(function(){try{var a=window.gbar;a.mcf(\"pm\",{p:\"\"});}catch(e){window.gbar&&gbar.logger&&gbar.logger.ml(e,{\"_sn\":\"cfg.init\"});}})();\n(function(){try{var a=window.gbar;a.mcf(\"mm\",{s:\"1\"});}catch(e){window.gbar&&gbar.logger&&gbar.logger.ml(e,{\"_sn\":\"cfg.init\"});}})();\n(function(){try{var d=window.gbar.i.i;var e=window.gbar;var f=e.i;var g=f.c(\"1\",0),h=/\\bgbmt\\b/,k=function(a){try{var b=document.getElementById(\"gb_\"+g),c=document.getElementById(\"gb_\"+a);b&&f.l(b,h.test(b.className)?\"gbm0l\":\"gbz0l\");c&&f.k(c,h.test(c.className)?\"gbm0l\":\"gbz0l\")}catch(l){d(l,\"sj\",\"ssp\")}g=a},m=e.qs,n=function(a){var b=a.href;var c=window.location.href.match(/.*?:\\/\\/[^\\/]*/)[0];c=new RegExp(\"^\"+c+\"/search\\\\?\");(b=c.test(b))&&!/(^|\\\\?|&)ei=/.test(a.href)&&(b=window.google)&&b.kEXPI&&(a.href+=\"&ei=\"+b.kEI)},p=function(a){m(a);\nn(a)},q=function(){if(window.google&&window.google.sn){var a=/.*hp$/;return a.test(window.google.sn)?\"\":\"1\"}return\"-1\"};e.rp=q;e.slp=k;e.qs=p;e.qsi=n;}catch(e){window.gbar&&gbar.logger&&gbar.logger.ml(e,{\"_sn\":\"cfg.init\"});}})();\n(function(){try{var a=this;var b=window.gbar;var c=b.i;var d=c.a,e=c.c,f={cty:\"USA\",cv:\"190405948\",dbg:d(\"\"),ecv:\"0\",ei:e(\"0yTMWv3UMeGN_QaribqQCQ\"),ele:d(\"1\"),esr:e(\"0.1\"),evts:[\"mousedown\",\"touchstart\",\"touchmove\",\"wheel\",\"keydown\"],gbl:\"es_plusone_gc_20180321.0_p0\",hd:\"com\",hl:\"en\",irp:d(\"\"),pid:e(\"1\"),\nsnid:e(\"28834\"),to:e(\"300000\"),u:e(\"\"),vf:\".66.41.\"},g=f,h=[\"bndcfg\"],k=a;h[0]in k||\"undefined\"==typeof k.execScript||k.execScript(\"var \"+h[0]);for(var l;h.length&&(l=h.shift());)h.length||void 0===g?k=k[l]&&k[l]!==Object.prototype[l]?k[l]:k[l]={}:k[l]=g;}catch(e){window.gbar&&gbar.logger&&gbar.logger.ml(e,{\"_sn\":\"cfg.init\"});}})();\n(function(){try{window.gbar.rdl();}catch(e){window.gbar&&gbar.logger&&gbar.logger.ml(e,{\"_sn\":\"cfg.init\"});}})();\n</script><link href=\"/images/branding/product/ico/googleg_lodp.ico\" rel=\"shortcut icon\"></head><body bgcolor=\"#fff\"><script nonce=\"MZUWGwd3D7nfH+HpDr55WA==\">(function(){var src='/images/nav_logo229.png';var iesg=false;document.body.onload = function(){window.n && window.n();if (document.images){new Image().src=src;}\nif (!iesg){document.f&&document.f.q.focus();document.gbqf&&document.gbqf.q.focus();}\n}\n})();</script><div id=\"mngb\"> <div id=gb><script>window.gbar&&gbar.eli&&gbar.eli()</script><div id=gbw><div id=gbz><span class=gbtcb></span><ol id=gbzc class=gbtc><li class=gbt><a onclick=gbar.logger.il(1,{t:1}); class=\"gbzt gbz0l gbp1\" id=gb_1 href=\"https://www.google.com/webhp?tab=ww\"><span class=gbtb2></span><span class=gbts>Search</span></a></li><li class=gbt><a onclick=gbar.logger.il(1,{t:2}); class=gbzt id=gb_2 href=\"http://www.google.com/imghp?hl=en&tab=wi\"><span class=gbtb2></span><span class=gbts>Images</span></a></li><li class=gbt><a onclick=gbar.logger.il(1,{t:8}); class=gbzt id=gb_8 href=\"http://maps.google.com/maps?hl=en&tab=wl\"><span class=gbtb2></span><span class=gbts>Maps</span></a></li><li class=gbt><a onclick=gbar.logger.il(1,{t:78}); class=gbzt id=gb_78 href=\"https://play.google.com/?hl=en&tab=w8\"><span class=gbtb2></span><span class=gbts>Play</span></a></li><li class=gbt><a onclick=gbar.logger.il(1,{t:36}); class=gbzt id=gb_36 href=\"http://www.youtube.com/?gl=US&tab=w1\"><span class=gbtb2></span><span class=gbts>YouTube</span></a></li><li class=gbt><a onclick=gbar.logger.il(1,{t:5}); class=gbzt id=gb_5 href=\"http://news.google.com/nwshp?hl=en&tab=wn\"><span class=gbtb2></span><span class=gbts>News</span></a></li><li class=gbt><a onclick=gbar.logger.il(1,{t:23}); class=gbzt id=gb_23 href=\"https://mail.google.com/mail/?tab=wm\"><span class=gbtb2></span><span class=gbts>Gmail</span></a></li><li class=gbt><a onclick=gbar.logger.il(1,{t:49}); class=gbzt id=gb_49 href=\"https://drive.google.com/?tab=wo\"><span class=gbtb2></span><span class=gbts>Drive</span></a></li><li class=gbt><a class=gbgt id=gbztm href=\"https://www.google.com/intl/en/options/\" onclick=\"gbar.tg(event,this)\" aria-haspopup=true aria-owns=gbd><span class=gbtb2></span><span id=gbztms class=\"gbts gbtsa\"><span id=gbztms1>More</span><span class=gbma></span></span></a><div class=gbm id=gbd aria-owner=gbztm><div id=gbmmb class=\"gbmc gbsb gbsbis\"><ol id=gbmm class=\"gbmcc gbsbic\"><li class=gbmtc><a onclick=gbar.logger.il(1,{t:24}); class=gbmt id=gb_24 href=\"https://www.google.com/calendar?tab=wc\">Calendar</a></li><li class=gbmtc><a onclick=gbar.logger.il(1,{t:51}); class=gbmt id=gb_51 href=\"http://translate.google.com/?hl=en&tab=wT\">Translate</a></li><li class=gbmtc><a onclick=gbar.logger.il(1,{t:17}); class=gbmt id=gb_17 href=\"http://www.google.com/mobile/?hl=en&tab=wD\">Mobile</a></li><li class=gbmtc><a onclick=gbar.logger.il(1,{t:10}); class=gbmt id=gb_10 href=\"https://books.google.com/bkshp?hl=en&tab=wp\">Books</a></li><li class=gbmtc><a onclick=gbar.logger.il(1,{t:6}); class=gbmt id=gb_6 href=\"http://www.google.com/shopping?hl=en&tab=wf\">Shopping</a></li><li class=gbmtc><a onclick=gbar.logger.il(1,{t:30}); class=gbmt id=gb_30 href=\"http://www.blogger.com/?tab=wj\">Blogger</a></li><li class=gbmtc><a onclick=gbar.logger.il(1,{t:27}); class=gbmt id=gb_27 href=\"http://www.google.com/finance?tab=we\">Finance</a></li><li class=gbmtc><a onclick=gbar.logger.il(1,{t:31}); class=gbmt id=gb_31 href=\"https://photos.google.com/?tab=wq&pageId=none\">Photos</a></li><li class=gbmtc><a onclick=gbar.logger.il(1,{t:12}); class=gbmt id=gb_12 href=\"http://video.google.com/?hl=en&tab=wv\">Videos</a></li><li class=gbmtc><a onclick=gbar.logger.il(1,{t:25}); class=gbmt id=gb_25 href=\"https://docs.google.com/document/?usp=docs_alc\">Docs</a></li><li class=gbmtc><div class=\"gbmt gbmh\"></div></li><li class=gbmtc><a onclick=gbar.logger.il(1,{t:66}); href=\"https://www.google.com/intl/en/options/\" class=gbmt>Even more &raquo;</a></li></ol><div class=gbsbt></div><div class=gbsbb></div></div></div></li></ol></div><div id=gbg><h2 class=gbxx>Account Options</h2><span class=gbtcb></span><ol class=gbtc><li class=gbt><a target=_top href=\"https://accounts.google.com/ServiceLogin?hl=en&passive=true&continue=http://www.google.com/\" onclick=\"gbar.logger.il(9,{l:'i'})\" id=gb_70 class=gbgt><span class=gbtb2></span><span id=gbgs4 class=gbts><span id=gbi4s1>Sign in</span></span></a></li><li class=\"gbt gbtb\"><span class=gbts></span></li><li class=gbt><a class=gbgt id=gbg5 href=\"http://www.google.com/preferences?hl=en\" title=\"Options\" onclick=\"gbar.tg(event,this)\" aria-haspopup=true aria-owns=gbd5><span class=gbtb2></span><span id=gbgs5 class=gbts><span id=gbi5></span></span></a><div class=gbm id=gbd5 aria-owner=gbg5><div class=gbmc><ol id=gbom class=gbmcc><li class=\"gbkc gbmtc\"><a  class=gbmt href=\"/preferences?hl=en\">Search settings</a></li><li class=gbmtc><div class=\"gbmt gbmh\"></div></li><li class=\"gbkp gbmtc\"><a class=gbmt href=\"http://www.google.com/history/optout?hl=en\">Web History</a></li></ol></div></div></li></ol></div></div><div id=gbx3></div><div id=gbx4></div><script>window.gbar&&gbar.elp&&gbar.elp()</script></div> </div><center><br clear=\"all\" id=\"lgpd\"><div id=\"lga\"><img alt=\"Google\" height=\"92\" src=\"/images/branding/googlelogo/1x/googlelogo_white_background_color_272x92dp.png\" style=\"padding:28px 0 14px\" width=\"272\" id=\"hplogo\" onload=\"window.lol&&lol()\"><br><br></div><form action=\"/search\" name=\"f\"><table cellpadding=\"0\" cellspacing=\"0\"><tr valign=\"top\"><td width=\"25%\">&nbsp;</td><td align=\"center\" nowrap=\"\"><input value=\"en\" name=\"hl\" type=\"hidden\"><input name=\"source\" type=\"hidden\" value=\"hp\"><input name=\"biw\" type=\"hidden\"><input name=\"bih\" type=\"hidden\"><div class=\"ds\" style=\"height:32px;margin:4px 0\"><input style=\"color:#000;margin:0;padding:5px 8px 0 6px;vertical-align:top\" autocomplete=\"off\" class=\"lst\" value=\"\" title=\"Google Search\" maxlength=\"2048\" name=\"q\" size=\"57\"></div><br style=\"line-height:0\"><span class=\"ds\"><span class=\"lsbb\"><input class=\"lsb\" value=\"Google Search\" name=\"btnG\" type=\"submit\"></span></span><span class=\"ds\"><span class=\"lsbb\"><input class=\"lsb\" value=\"I'm Feeling Lucky\" name=\"btnI\" onclick=\"if(this.form.q.value)this.checked=1; else top.location='/doodles/'\" type=\"submit\"></span></span></td><td class=\"fl sblc\" align=\"left\" nowrap=\"\" width=\"25%\"><a href=\"/advanced_search?hl=en&amp;authuser=0\">Advanced search</a><a href=\"/language_tools?hl=en&amp;authuser=0\">Language tools</a></td></tr></table><input id=\"gbv\" name=\"gbv\" type=\"hidden\" value=\"1\"><script nonce=\"MZUWGwd3D7nfH+HpDr55WA==\">(function(){var a,b=\"1\";if(document&&document.getElementById)if(\"undefined\"!=typeof XMLHttpRequest)b=\"2\";else if(\"undefined\"!=typeof ActiveXObject){var c,d,e=[\"MSXML2.XMLHTTP.6.0\",\"MSXML2.XMLHTTP.3.0\",\"MSXML2.XMLHTTP\",\"Microsoft.XMLHTTP\"];for(c=0;d=e[c++];)try{new ActiveXObject(d),b=\"2\"}catch(h){}}a=b;if(\"2\"==a&&-1==location.search.indexOf(\"&gbv=2\")){var f=google.gbvu,g=document.getElementById(\"gbv\");g&&(g.value=a);f&&window.setTimeout(function(){location.href=f},0)};}).call(this);</script></form><div id=\"gac_scont\"></div><div style=\"font-size:83%;min-height:3.5em\"><br></div><span id=\"footer\"><div style=\"font-size:10pt\"><div style=\"margin:19px auto;text-align:center\" id=\"fll\"><a href=\"/intl/en/ads/\">Advertising Programs</a><a href=\"/services/\">Business Solutions</a><a href=\"https://plus.google.com/116899029375914044550\" rel=\"publisher\">+Google</a><a href=\"/intl/en/about.html\">About Google</a></div></div><p style=\"color:#767676;font-size:8pt\">&copy; 2018 - <a href=\"/intl/en/policies/privacy/\">Privacy</a> - <a href=\"/intl/en/policies/terms/\">Terms</a></p></span></center><script nonce=\"MZUWGwd3D7nfH+HpDr55WA==\">(function(){window.google.cdo={height:0,width:0};(function(){var a=window.innerWidth,b=window.innerHeight;if(!a||!b){var c=window.document,d=\"CSS1Compat\"==c.compatMode?c.documentElement:c.body;a=d.clientWidth;b=d.clientHeight}a&&b&&(a!=google.cdo.width||b!=google.cdo.height)&&google.log(\"\",\"\",\"/client_204?&atyp=i&biw=\"+a+\"&bih=\"+b+\"&ei=\"+google.kEI);}).call(this);})();</script><div id=\"xjsd\"></div><div id=\"xjsi\"><script nonce=\"MZUWGwd3D7nfH+HpDr55WA==\">(function(){function c(b){window.setTimeout(function(){var a=document.createElement(\"script\");a.src=b;google.timers&&google.timers.load.t&&google.tick(\"load\",{gen204:\"xjsls\",clearcut:31});document.getElementById(\"xjsd\").appendChild(a)},0)}google.dljp=function(b,a){google.xjsu=b;c(a)};google.dlj=c;}).call(this);if(!google.xjs){window._=window._||{};window._DumpException=window._._DumpException=function(e){throw e};window._F_installCss=window._._F_installCss=function(c){};google.dljp('/xjs/_/js/k\\x3dxjs.hp.en_US.iwMXH3MSrcU.O/m\\x3dsb_he,d/am\\x3dVDA2/rt\\x3dj/d\\x3d1/t\\x3dzcms/rs\\x3dACT90oHMjB_NKgQtPI3KVLNuNBuyDaD8iA','/xjs/_/js/k\\x3dxjs.hp.en_US.iwMXH3MSrcU.O/m\\x3dsb_he,d/am\\x3dVDA2/rt\\x3dj/d\\x3d1/t\\x3dzcms/rs\\x3dACT90oHMjB_NKgQtPI3KVLNuNBuyDaD8iA');google.xjs=1;}google.pmc={\"sb_he\":{\"agen\":true,\"cgen\":true,\"client\":\"heirloom-hp\",\"dh\":true,\"dhqt\":true,\"ds\":\"\",\"ffql\":\"en\",\"fl\":true,\"host\":\"google.com\",\"isbh\":28,\"jsonp\":true,\"msgs\":{\"cibl\":\"Clear Search\",\"dym\":\"Did you mean:\",\"lcky\":\"I\\u0026#39;m Feeling Lucky\",\"lml\":\"Learn more\",\"oskt\":\"Input tools\",\"psrc\":\"This search was removed from your \\u003Ca href=\\\"/history\\\"\\u003EWeb History\\u003C/a\\u003E\",\"psrl\":\"Remove\",\"sbit\":\"Search by image\",\"srch\":\"Google Search\"},\"nds\":true,\"ovr\":{},\"pq\":\"\",\"refpd\":true,\"rfs\":[],\"sbpl\":24,\"sbpr\":24,\"scd\":10,\"sce\":5,\"stok\":\"FQhoPz-jwOPoIaPtd4-yNKW5coU\"},\"d\":{},\"ZI/YVQ\":{},\"U5B21g\":{},\"DPBNMg\":{},\"YFCs/g\":{}};google.x(null,function(){});(function(){var r=[];google.plm(r);})();(function(){var ctx=[]\n;google.jsc && google.jsc.x(ctx);})();</script></div></body></html>\n"
  # "The script will output this if it catches a HTTP Error."
  # "$request =\ntry { \n    Invoke-WebRequest httpbin.org/get\n    $err = 'false'\n} catch {\n    $_.exception\n    $errorresponse = $error[0].errordetails.message\n    $err = 'true'\n    $errorresponse\n}\nif ($err -eq 'false') {\n    $request.rawcontent\n} else {\n    $request\n}"
  n1 = Match Pattern(string="HTTP Response", regular expression="The remote server returned an error:") -> (match substring=w4:string)  [unwired: 1 in, 3 out]
  n2 = Empty String/Path?(string/path=w4) -> (empty?=w3:bool)
  n3 = case shown="True" w3 {
    tunnel: [w19 w45] -> w11
    tunnel: [w13 w43] -> w10
    tunnel: "HTTP Response" -> [w22 w42]
    tunnel: [w14 w38] -> w9
    tunnel: ["" w40] -> w8
    tunnel: [w20 w32] -> w7
    tunnel: [cluster{"Name":string, "Value":string}[] [] w41] -> w6
    frame False {
      # "Get rid of parenthesis, periods, and other special characters that shouldnt be in the status description (because of the way that PowerShell Handles Errors)"
      # "Search for the status code"
      # "Specific to the scripts I've created"
      n4 = Match Pattern(string=w22, regular expression="\\n") -> (before substring=w19:string, after substring=w20:string)  [unwired: 1 in, 2 out]
      n5 = Match Pattern(string=w19, regular expression="[1-5][0-9][0-9]") -> (match substring=w13:string, after substring=w12:string)  [unwired: 1 in, 2 out]
      n6 = while {
        tunnel: [w28] -> w15 mode=indexing
        shift-right: [w25] -> _
        shift-left: w12 -> [w29]
        tunnel: "[A-Z a-z 0-9]" ("search string") -> [w24]
        stop <- w26 stop-if-true
        n7 = Match Pattern(string=w29, regular expression=w24) -> (match substring=w28:string, after substring=w25:string, offset past match=w27:i32)  [unwired: 1 in, 1 out]
        n8 = Less Than 0?(x=w27) -> (x < 0?=w26:bool)
      }
      n9 = Concatenate Strings(w15) -> (w14:string)
    }
    frame True {
      (unwired) "[\\r\\n][\\r\\n]" ("regular expression")
      # "https://stackoverflow.com/questions/8474745/how-do-i-get-the-body-of-a-http-response-from-a-string-containing-the-entire-res\n\nThis goes into some detail why i have to have this case structure to atttempt to parse the response again. It is under the question, update 3"
      # "Turn the headers into an array of Name, Value pairs"
      # "Regex for <enter>\nSeperating out the status line from the headers"
      # "Regex for empty line.\nSplits up the headers from the body"
      # "Regex for status code"
      n10 = Match Pattern(string=w42, regular expression="\\n") -> (before substring=w45:string, after substring=w46:string)  [unwired: 1 in, 2 out]
      n11 = call <vilib>:"Trim Whitespace.vi"("string"=w46) -> ("trimmed string"=w37:string)  [unwired: 1 in]
      n12 = Match Pattern(string=w37, regular expression="\\n\\n") -> (before substring=w33:string, match substring=w36:string, after substring=w35:string)  [unwired: 1 in, 1 out]
      n13 = Empty String/Path?(string/path=w36) -> (empty?=w34:bool)
      n14 = case shown="False" w34 {
        tunnel: w35 -> [w48 _]
        tunnel: w33 -> [w49 w50]
        tunnel: [w48 w52] -> w32
        tunnel: [w49 w51] -> w31
        frame False {
        }
        frame True {
          n15 = Match Pattern(string=w50, regular expression="\\r\\n\\r\\n") -> (before substring=w51:string, after substring=w52:string)  [unwired: 1 in, 2 out]
        }
      }
      n16 = Match Pattern(string=w45, regular expression="[1-5][0-9][0-9]") -> (before substring=w40:string, match substring=w43:string, after substring=w39:string)  [unwired: 1 in, 1 out]
      n17 = while {
        tunnel: [w63] -> w41 mode=indexing
        shift-right: [w55] -> _
        shift-left: w31 -> [w60]
        stop <- w61 stop-if-true
        n18 = Match Pattern(string=w60, regular expression="\\n") -> (before substring=w66:string, after substring=w55:string)  [unwired: 1 in, 2 out]
        n19 = call <vilib>:"Trim Whitespace.vi"("string"=w55) -> ("trimmed string"=w54:string)  [unwired: 1 in]
        n20 = Match Pattern(string=w66, regular expression=":") -> (before substring=w59:string, after substring=w57:string)  [unwired: 1 in, 2 out]
        n21 = String Length(string=w54) -> (length=w62:i32)
        n22 = call <vilib>:"Trim Whitespace.vi"("string"=w59) -> ("trimmed string"=w58:string)  [unwired: 1 in]
        n23 = call <vilib>:"Trim Whitespace.vi"("string"=w57) -> ("trimmed string"=w56:string)  [unwired: 1 in]
        n24 = Equal To 0?(x=w62) -> (x = 0?=w61:bool)
        n25 = Bundle(cluster=cluster{"Name":string, "Value":string} {"Name"="", "Value"=""}, "Name"=w58, "Value"=w56) -> (w63:cluster{"Name":string, "Value":string})
      }
      n26 = call <vilib>:"Trim Whitespace.vi"("string"=w39) -> ("trimmed string"=w38:string)  [unwired: 1 in]
    }
  }
  "Status Line" <- w11
  "Body" <- w7
  "Status Description" <- w9
  "Protocol" <- w8
  "Headers" <- w6
  "Status Code" <- w10
  "error out" <- "error in (no error)"
